vi "lv flush buffer to stream.vi"(8 "error in":errorcluster, 11 "buffer handle":i32) -> (0 "error out":errorcluster)   [LabVIEW 2026]
uses:
  lv deref string.vi
  <vilib>/Utility/error.llb/Error Cluster From Error Code.vi
  bin/nominalClient_64.dll
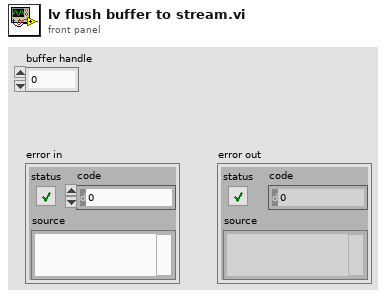
[diagram p1: front panel]
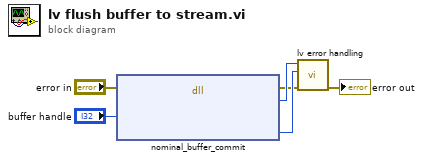
[diagram p0: block diagram]
diagram:
  n1 = dll-call lib="C:/sw/nominal-c/bin/nominalClient_64.dll" fn="nominal_buffer_commit"(error in="error in", "buffer"="buffer handle") -> (error out=w3:errorcluster, "return type"=w4:i32, "errorout"=w5:i32)  [unwired: 4 in, 1 out]
  n2 = call "lv error handling.vi"("error in"=w3, "error handle"=w5, "return code"=w4) -> ("error out"=→"error out":errorcluster)  [unwired: 8 in]
